vi "Motor2CableMismatch.vi"(7 "TotalMotorNumber":i32=8, 8 "CableTension":dbl[](array[numeric]), 11 "Cable#":i32[](array[numeric])) -> (0 "MotorTension":dbl[](array[numeric]))   [LabVIEW 2015]
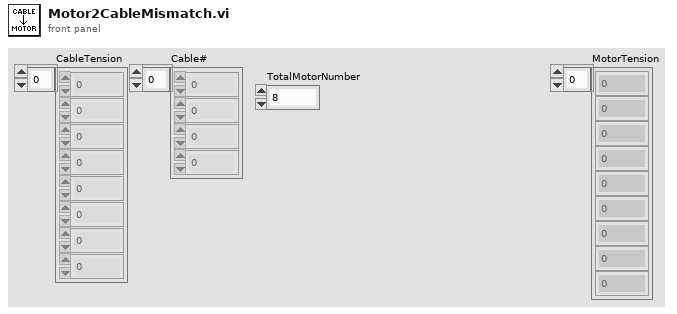
[diagram p1: front panel]
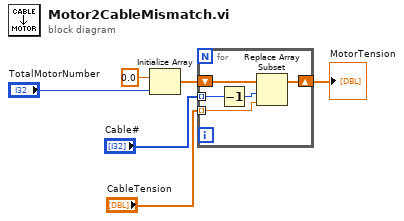
[diagram p0: block diagram]
diagram:
  n1 = Initialize Array(0.0 ("element"), "TotalMotorNumber") -> (w4:dbl[])
  n2 = for {
    tunnel: "CableTension" -> [w9] mode=indexing
    tunnel: "Cable#" -> [w10] mode=indexing
    shift-right: [w7] -> w1
    shift-left: w4 -> [w11]
    n3 = Decrement(x=w10) -> (x-1=w8:i32)
    n4 = Replace Array Subset(array=w11, new element=w9, index=w8) -> (w7:dbl[])
  }
  "MotorTension" <- w1
